vi "python_integration_computer_vision.vi"() -> ()   [LabVIEW 2022 SP3]
panel:
  out "return value":string
  in  "error in (no error)":errorcluster
  out "error out":errorcluster
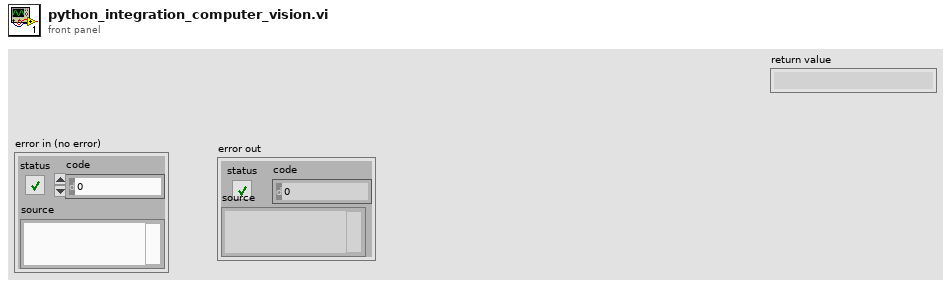
[diagram p1: front panel]
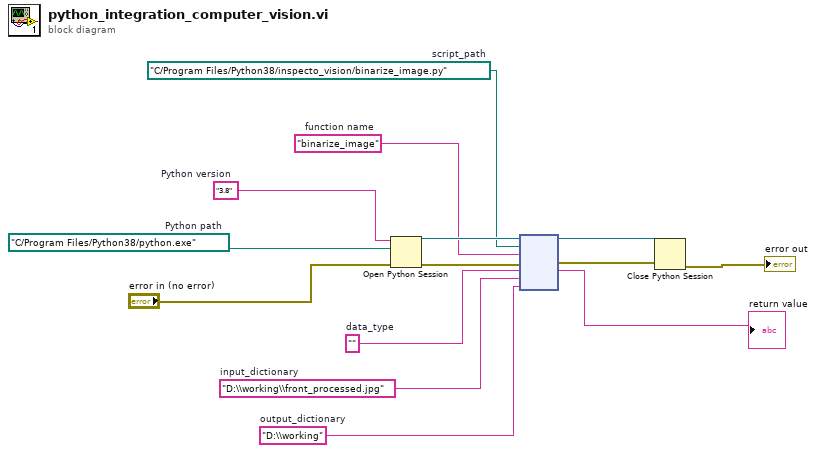
[diagram p0: block diagram]
diagram:
  w2 = "D:\\working"  # output_dictionary
  w3 = "D:\\working\\front_processed.jpg"  # input_dictionary
  w4 = ""  # data_type
  w5 = "binarize_image"  # function name
  w6 = path "C:/Program Files/Python38/inspecto_vision/binarize_image.py"  # script_path
  w8 = path "C:/Program Files/Python38/python.exe"  # Python path
  w9 = "3.8"  # Python version
  n1 = Open Python Session(python version=w9, python path=w8, 3:"error in (no error)") -> (session out=w13:refnum<k35>, error out=w12:errorcluster)
  n2 = node(w13, w6, w5, w12, w4, w3, w2) -> (w14:refnum<k35>, w11:errorcluster, →"return value":string)  [unwired: 2 in, 2 out]
  n3 = Close Python Session(session in=w14, error in=w11) -> (11:→"error out":errorcluster)
